vi "测量伏安特性.vi"() -> ()   [LabVIEW 2014]
uses:
  <vilib>/Analysis/NI_AALPro.lvlib
panel:
  out "数据":dbl[][](array[numeric])
  out "待测电阻阻值":dbl
  in  "标准电阻":dbl
  in  "测量数据点数":dbl
  in  "时间间隔":dbl[unit]
  in  "电压步长":dbl[unit]
  out "伏安特性曲线":cluster{"Y":dbl[], "Y":dbl[]}[](graph)
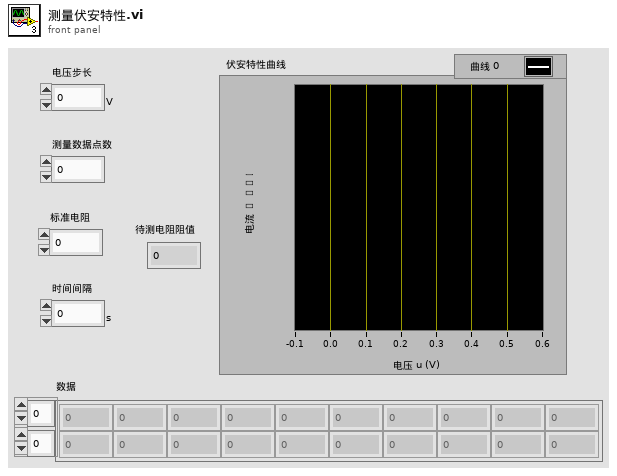
[diagram p1: front panel]
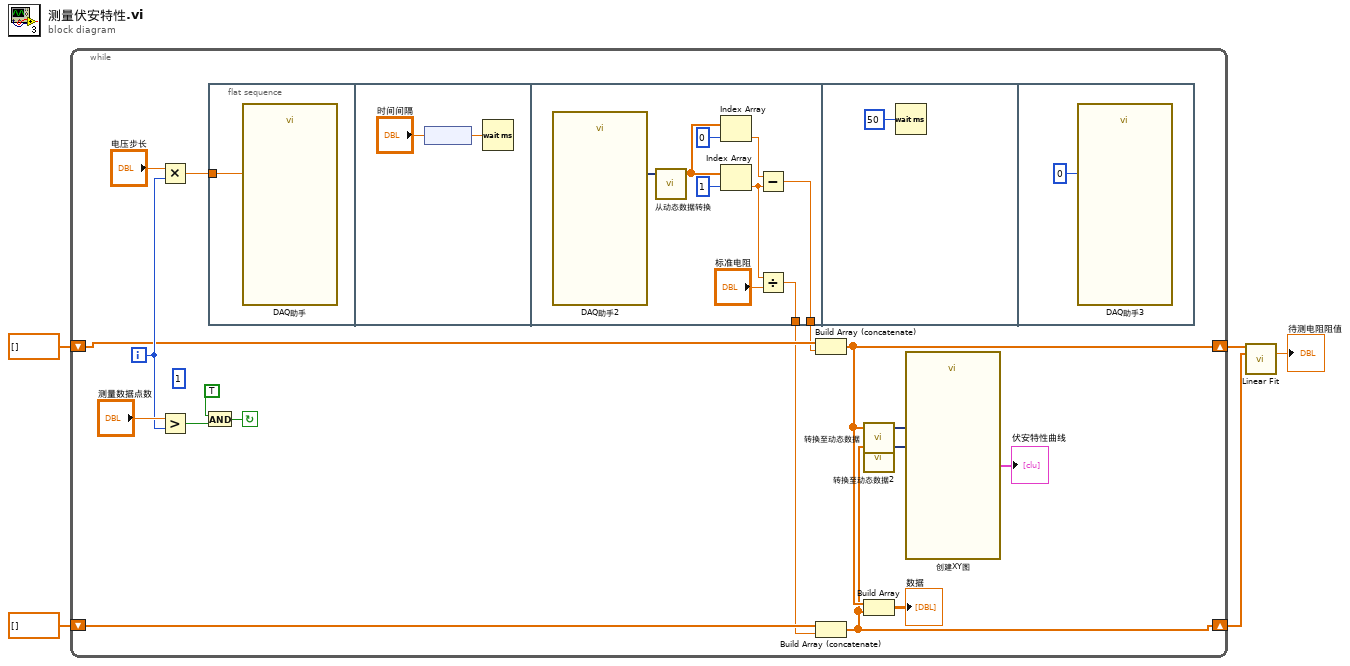
[diagram p0: block diagram]
diagram:
  n1 = while {
    shift-right: [w10] -> w2
    shift-left: dbl[] [] -> [w15]
    shift-right: [w8] -> w3
    shift-left: dbl[] [] -> [w14]
    i -> [w18]
    stop <- w16 continue-if-true
    (unwired) 1
    n2 = Multiply(x="电压步长", y=w18) -> (x*y=w20:dbl[unit])
    n3 = Greater?(x="测量数据点数", y=w18) -> (0:w17:bool)
    n4 = And(x=TRUE, y=w17) -> (x .and. y?=w16:bool)
    n5 = flat-sequence {
      tunnel: w20 -> [w23]
      tunnel: [w27] -> w13
      tunnel: [w26] -> w12
      frame #0 {
        n6 = call "DAQ助手"("data"=w23) -> ()  [unwired: 17 in, 2 out]
      }
      frame #1 {
        n7 = node("时间间隔") -> (w24:dbl)
        n8 = Wait (ms)(milliseconds to wait=w24) -> ()  [unwired: 1 out]
      }
      frame #2 {
        n9 = call "DAQ助手2"() -> ("data"=w34:dynamicdata)  [unwired: 17 in, 2 out]
        n10 = call "从动态数据转换"("Dynamic Data Type"=w34) -> ("Array"=w33:dbl[])  [unwired: 3 in]
        n11 = Index Array(array=w33, index=0 ("索引")) -> (element=w30:dbl)
        n12 = Index Array(array=w33, index=1 ("索引")) -> (element=w29:dbl)
        n13 = Subtract(x=w30, y=w29) -> (x-y=w27:dbl)
        n14 = Divide(x=w29, y="标准电阻") -> (x/y=w26:dbl)
      }
      frame #3 {
        n15 = Wait (ms)(milliseconds to wait=50) -> ()  [unwired: 1 out]
      }
      frame #4 {
        n16 = call "DAQ助手3"("data"=0) -> ()  [unwired: 17 in, 2 out]
      }
    }
    n17 = Build Array (concatenate)(w15, w13) -> (w10:dbl[])
    n18 = Build Array (concatenate)(w14, w12) -> (w8:dbl[])
    n19 = call "转换至动态数据"("Array"=w10) -> ("Dynamic Data Type"=w9:dynamicdata)  [unwired: 3 in]
    n20 = call "转换至动态数据2"("Array"=w8) -> ("Dynamic Data Type"=w7:dynamicdata)  [unwired: 3 in]
    n21 = Build Array(w10, w8) -> (→"数据":dbl[][])
    n22 = call "创建XY图"("Y Input"=w7, "X Input"=w9) -> ("XY Graph"=→"伏安特性曲线":cluster{"X":dbl[], "Y":dbl[]}[])  [unwired: 8 in, 1 out]
  }
  n23 = call <vilib>:"Linear Fit.vi"("Y"=w2, "X"=w3) -> ("slope"=→"待测电阻阻值":dbl)  [unwired: 9 in, 4 out]
